vi "CoordinateConvert_ShoulderOriginCartesianToWorldCartesian.vi"(1 "ArmPositionRelativeToShoulderIn":T1, 2 "RobotDimensions":T2) -> (0 "ArmPosition":T1)   [LabVIEW 2018]
uses:
  TypeDefs/ConfigComponents/Config_Dimensions.ctl
  TypeDefs/ArmAbsolutePosition.ctl
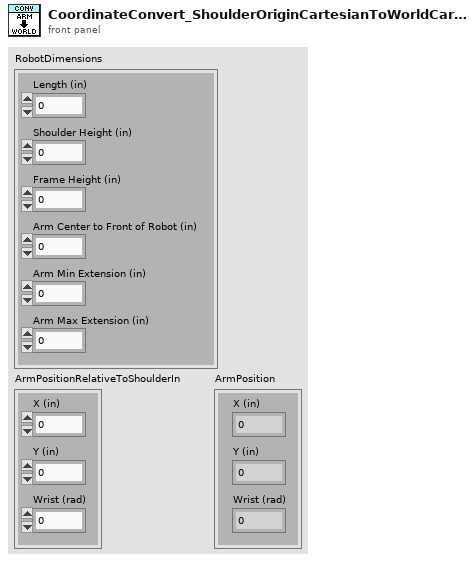
[diagram p1: front panel]
types:
  T1 = typedef "ArmAbsolutePosition.ctl" = cluster{"X (in)":dbl, "Y (in)":dbl, "Wrist (rad)":dbl}
  T2 = typedef "Config_Dimensions.ctl" = cluster{"Length (in)":dbl, "Shoulder Height (in)":dbl, "Frame Height (in)":dbl, "Arm Center to Front of Robot (in)":dbl, "Arm Min Extension (in)":dbl, "Arm Max Extension (in)":dbl}
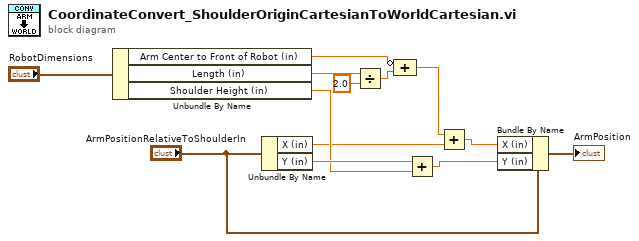
[diagram p0: block diagram]
diagram:
  n1 = Unbundle By Name("RobotDimensions") -> ("Arm Center to Front of Robot (in)"=w9:dbl, "Length (in)"=w11:dbl, "Shoulder Height (in)"=w6:dbl)
  n2 = Unbundle By Name("ArmPositionRelativeToShoulderIn") -> ("X (in)"=w3:dbl, "Y (in)"=w7:dbl)
  n3 = Divide(x=w11, y=2.0) -> (x/y=w8:dbl)
  n4 = Compound Arithmetic op=ADD(invert w9, w8) -> (w4:dbl)
  n5 = Add(x=w7, y=w6) -> (x+y=w5:dbl)
  n6 = Add(x=w4, y=w3) -> (x+y=w2:dbl)
  n7 = Bundle By Name(cluster="ArmPositionRelativeToShoulderIn", "X (in)"=w2, "Y (in)"=w5) -> (→"ArmPosition":T1)
